vi "Load Device Channels.vi"(8 "Error In":errorcluster, 11 "Device Config":T1) -> (0 "Error Out":errorcluster, 3 "Device Config":T1)   [LabVIEW 2020, in "LMH-LINX.lvlib" / "myRIO.lvlib"]
uses:
  myRIO.lvlib
  Device/Type Defs/LINX Device Config.ctl
  Type Defs/Interface.ctl
  Device/Type Defs/TCP Config.ctl
  Device/Type Defs/Channels.ctl
  Type Defs/Error Type.ctl
  LMH-LINX.lvlib
  Device/Device.lvlib
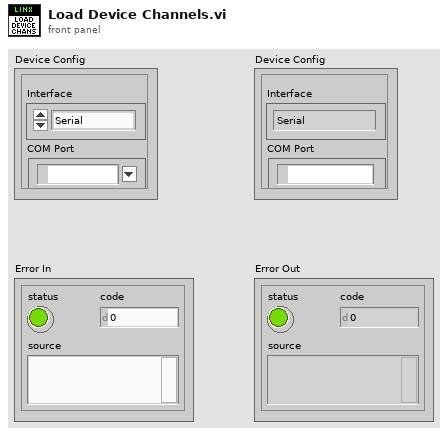
[diagram p1: front panel]
types:
  T1 = typedef "LMH-LINX.lvlib/Device.lvlib/LINX Device Config.ctl" = cluster{"Interface":T2, "COM Port":refnum<visa-resource-name>, "TCP Configuration":T3, "Device Family":u8, "Device ID":u8, "Device Name":string, "TCP Ref":refnum<k5>, "Channels":T4}
  T2 = typedef "LMH-LINX.lvlib/Interface.ctl" = enum16{"Serial", "TCP"}
  T3 = typedef "LMH-LINX.lvlib/Device.lvlib/TCP Config.ctl" = cluster{"IP Address":string, "Port":u16}
  T4 = typedef "LMH-LINX.lvlib/Channels.ctl" = cluster{"DI":u8[], "DO":u8[], "AI":u8[], "AO":u8[], "PWM":u8[], "QE":u8[], "UART":u8[], "I2C 2":u8[], "SPI":u8[], "CAN":u8[], "Servo":u8[], "AI Ref (V)":dbl, "AI Resolution (Bits)":u8, "AO Ref (V)":dbl, "AO Resolution (Bits)":u8}
  T5 = typedef "LMH-LINX.lvlib/Error Type.ctl" = enum16{"Unknown", "Timeout", "Corrupt Return Packet", "Unable To Connect", "Command Not Supported", "Channel DNE", "Invalid COM Config", "Firmware Version Mismatch", "myRIO Support", "CMD Specific Error", "Local IO Not Supported"}
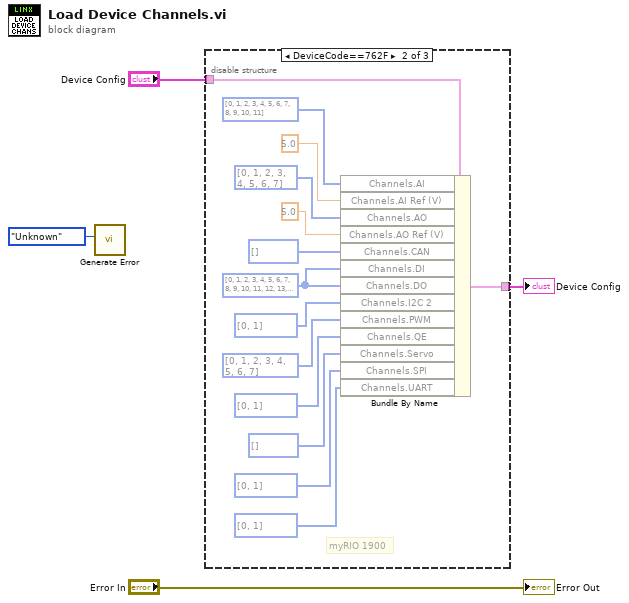
[diagram p0: block diagram]
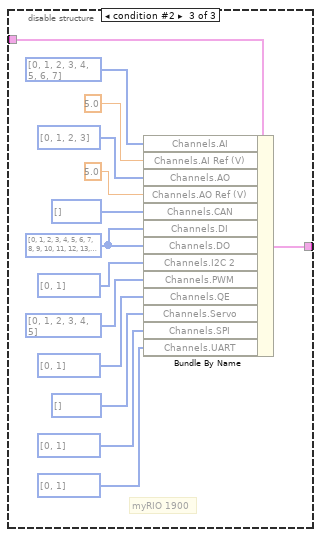
[diagram p3: hidden frame]
diagram:
  n1 = call "Generate Error.vi"("Error Type"=Error_Type."Unknown") -> ()  [unwired: 9 in, 2 out]
  n2 = disable-structure shown="DeviceCode==762F" {
    disable-tunnel: [w5 w7 w21] -> w4
    disable-tunnel: "Device Config" -> [w5 w6 w20]
    frame condition #0 (active) {
    }
    frame condition #1 {
      w19 = u8[] [0, 1, 2, 3, 4, 5, 6, 7, 8, 9, 10, 11, 12, 13, 14, 15, 16, 17, 18, 19, 20, 21, 22, 23, 24, 25, 26, 27, 28, 29, 30, 31, 32, 33, 34, 35, 36, 37, 38, 39, 0] ("myRIO-1900 Digital")
      # "myRIO 1900"
      n3 = Bundle By Name(cluster=w6, "Channels.AI"=u8[] [0, 1, 2, 3, 4, 5, 6, 7, 8, 9, 10, 11], "Channels.AI Ref (V)"=5.0, "Channels.AO"=u8[] [0, 1, 2, 3, 4, 5, 6, 7], "Channels.AO Ref (V)"=5.0, "Channels.CAN"=u8[] [], "Channels.DI"=w19, "Channels.DO"=w19, "Channels.I2C 2"=u8[] [0, 1], "Channels.PWM"=u8[] [0, 1, 2, 3, 4, 5, 6, 7], "Channels.QE"=u8[] [0, 1] ("Channels.I2C 2"), "Channels.Servo"=u8[] [], "Channels.SPI"=u8[] [0, 1] ("Channels.I2C 2"), "Channels.UART"=u8[] [0, 1] ("Channels.I2C 2")) -> (w7:T1)
    }
    frame condition #2 {
      w33 = u8[] [0, 1, 2, 3, 4, 5, 6, 7, 8, 9, 10, 11, 12, 13, 14, 15, 16, 17, 18, 19, 20, 21, 22, 23, 24, 25, 26, 27, 28, 29, 30, 31, 0] ("myRIO-1900 Digital")
      # "myRIO 1900"
      n4 = Bundle By Name(cluster=w20, "Channels.AI"=u8[] [0, 1, 2, 3, 4, 5, 6, 7], "Channels.AI Ref (V)"=5.0, "Channels.AO"=u8[] [0, 1, 2, 3], "Channels.AO Ref (V)"=5.0, "Channels.CAN"=u8[] [], "Channels.DI"=w33, "Channels.DO"=w33, "Channels.I2C 2"=u8[] [0, 1], "Channels.PWM"=u8[] [0, 1, 2, 3, 4, 5], "Channels.QE"=u8[] [0, 1] ("Channels.I2C 2"), "Channels.Servo"=u8[] [], "Channels.SPI"=u8[] [0, 1] ("Channels.I2C 2"), "Channels.UART"=u8[] [0, 1] ("Channels.I2C 2")) -> (w21:T1)
    }
  }
  "Device Config" <- w4
  "Error Out" <- "Error In"
